vi "Entry.vi"(8 "error in (no error)":errorcluster, 11 "New State":refnum<class "GTH-Down.lvclass">) -> (0 "error out":errorcluster, 3 "State out":refnum<class "GTH-Down.lvclass">)   [LabVIEW 2014, in "Elevator.lvlib" / "EL-Go To Height.lvlib" / "GTH-Down.lvclass"]
doc: "This is an abstract method. Override this method to define the behavior when you enter the state."
uses:
  GTH-Down.lvclass
  Elevator Messages/Set Rate (Percent) Msg/Set Rate (Percent) Msg.lvclass/Set Rate (Percent) Msg.ctl
  <vilib>/ActorFramework/Message Enqueuer/Message Enqueuer.lvclass/Message Enqueuer.ctl
  <vilib>/ActorFramework/Message Enqueuer/Enqueue.vi
  <vilib>/ActorFramework/Message Priority Queue/Priority Enqueue.vi
  EL-Go To Height Class/EL-Go To Height.lvclass
  Elevator Messages/Set Rate (Percent) Msg/Set Rate (Percent) Msg.lvclass
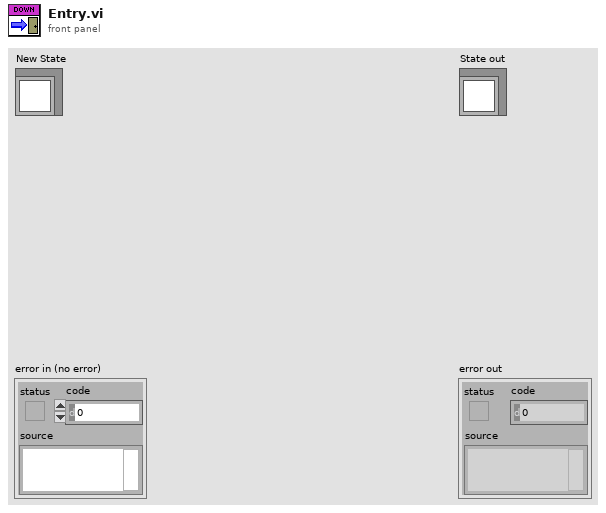
[diagram p1: front panel]
types:
  T1 = typedef "Elevator.lvlib/EL-Go To Height.lvlib/EL-Go To Height.lvclass/Parameters.ctl" = cluster{"Target Height":dbl, "Elevator State Loop (ms)":u32, "Up Rate (Percentage)":dbl, "Down Rate (Percentage)":dbl}
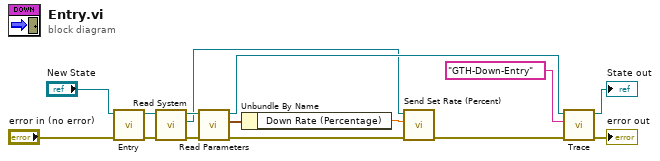
[diagram p0: block diagram]
diagram:
  n1 = call-parent "Entry.vi"("error in (no error)"="error in (no error)", "New State"="New State") -> ("error out"=w5:errorcluster, "State out"=w13:refnum<class "GTH-Down.lvclass">)  [unwired: 8 in]
  n2 = call-dynamic "Read System.vi"("error in (no error)"=w5, "Command in"=w13) -> ("error out"=w4:errorcluster, "Actor Framework:Message Enqueuer"=w8:refnum<class "Message Enqueuer.lvclass">, "Command out"=w12:refnum<class "GTH-Down.lvclass">)  [unwired: 7 in]
  n3 = call-dynamic "Read Parameters.vi"("error in (no error)"=w4, "EL-Go To Height in"=w12) -> ("error out"=w3:errorcluster, "Parameters"=w7:T1, "EL-Go To Height out"=w11:refnum<class "GTH-Down.lvclass">)  [unwired: 7 in]
  n4 = Unbundle By Name(w7) -> ("Down Rate (Percentage)"=w6:dbl)
  n5 = call "Send Set Rate (Percent).vi"("error in (no error)"=w3, "Percent"=w6, "Message Enqueuer"=w8) -> ("error out"=w2:errorcluster)  [unwired: 7 in, 1 out]
  n6 = call-dynamic "Trace.vi"("error in (no error)"=w2, "Command Action"="GTH-Down-Entry", "Command Actor in"=w11) -> ("error out"=→"error out":errorcluster, "Command Actor out"=→"State out":refnum<class "GTH-Down.lvclass">)  [unwired: 7 in]
